vi "StarTrekIndicator.vi"(4 "in":bool[](array[boolean])) -> (1 "out":bool[](array[boolean]))   [LabVIEW 2016, in "Instrument.OxfordVRM UI.lvclass"]
uses:
  Instrument.OxfordVRM UI.lvclass
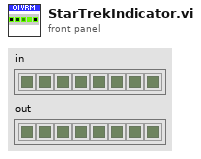
[diagram p1: front panel]
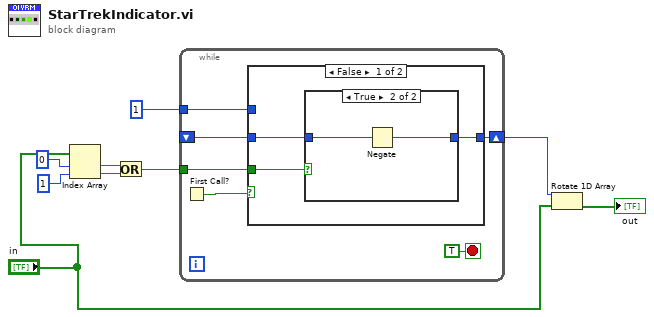
[diagram p0: block diagram]
diagram:
  n1 = Index Array(array="in", index #1=0 ("index"), index #2=1 ("index")) -> (element #1=w5:bool, element #2=w6:bool)
  n2 = Or(x=w5, y=w6) -> (x .or. y?=w4:bool)
  n3 = while {
    shift-right: [w10] -> w2
    shift-left: _ -> [w13]
    tunnel: w4 -> [w14]
    tunnel: 1 ("n") -> [w11]
    stop <- TRUE stop-if-true
    n4 = First Call?() -> (First Call?: T/F=w12:bool)
    n5 = case shown="False" w12 {
      tunnel: w14 -> [w18 _]
      tunnel: w13 -> [w17 _]
      tunnel: w11 -> [_ w22]
      tunnel: [w16 w22] -> w10
      frame False {
        n6 = case shown="True" w18 {
          tunnel: w17 -> [w19 w21]
          tunnel: [w19 w20] -> w16
          frame False {
          }
          frame True {
            n7 = Negate(x=w21) -> (-x=w20:i32)
          }
        }
      }
      frame True {
      }
    }
  }
  n8 = Rotate 1D Array(1:"in", 2:w2) -> (0:→"out":bool[])
